vi "ANC300_Input.vi"(0 "ANC300 Communication Port In":refnum<visa-resource-name>, 1 "connection ID in":refnum<k5>, 2 "Axis":u8=1 min=1 max=7, 3 "ON / OFF":bool=TRUE, 4 "AC / DC":bool=TRUE, 5 "error in":T1, 7 "Time to wait [ms]":u32=200, 8 "set / get":bool=TRUE) -> (13 "command string":string, 14 "ANC300 Communication Port Out":refnum<visa-resource-name>, 15 "connection ID out":refnum<k5>, 16 "transfer ok":bool, 17 "ON / OFF":bool=TRUE, 18 "data out":string, 19 "error out":T1)   [LabVIEW 2022 SP3]
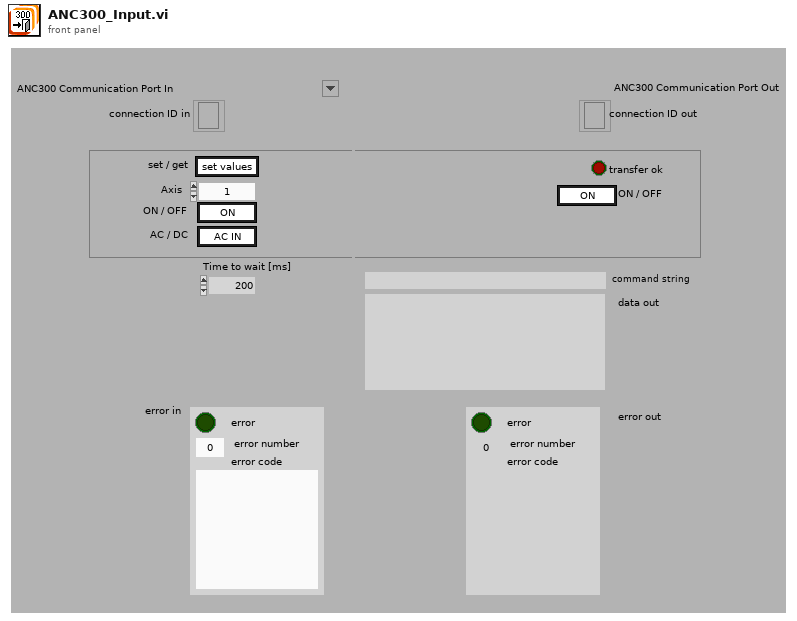
[diagram p1: front panel]
types:
  T1 = cluster{"error ":bool, "error number":i32, "error code":string}
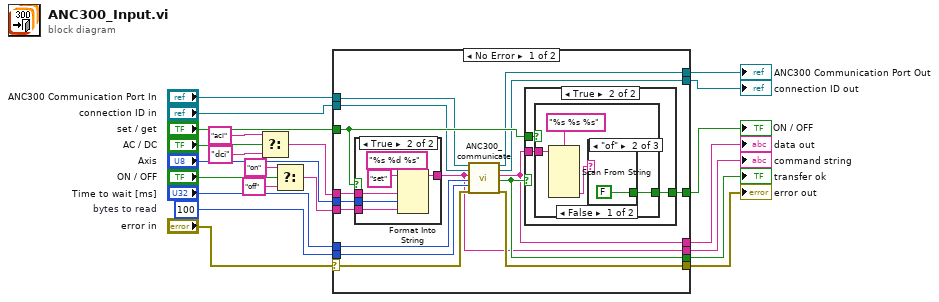
[diagram p0: block diagram]
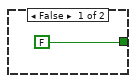
[diagram p2: hidden frame]
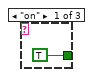
[diagram p3: hidden frame]
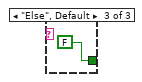
[diagram p4: hidden frame]
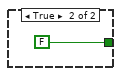
[diagram p5: hidden frame]
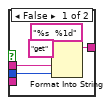
[diagram p6: hidden frame]
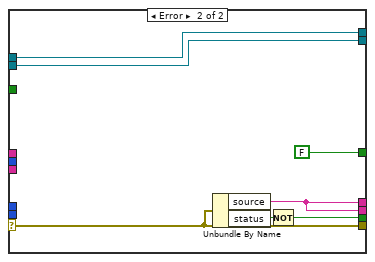
[diagram p7: hidden frame]
diagram:
  w17 = 100  # bytes to read
  n1 = Select(t="aci", s="AC / DC", f="dci") -> (s? t:f=w2:string)
  n2 = Select(t="on", s="ON / OFF", f="off") -> (s? t:f=w3:string)
  n3 = case shown="No Error" "error in" {
    selector: "error in" -> [w26 w66]
    tunnel: w2 -> [w38 _]
    tunnel: "Axis" -> [w37 _]
    tunnel: w3 -> [w36 _]
    tunnel: "set / get" -> [w35 _]
    tunnel: "ANC300 Communication Port In" -> [w34 w68]
    tunnel: "connection ID in" -> [w33 w67]
    tunnel: "Time to wait [ms]" -> [w32 _]
    tunnel: w17 -> [w31 _]
    tunnel: [w30 FALSE] -> w1
    tunnel: [w29 w66] -> w11
    tunnel: [w28 w68] -> w15
    tunnel: [w27 w67] -> w14
    tunnel: [w25 w64] -> w10
    tunnel: [w24 w63] -> w13
    tunnel: [w23 w63] -> w12
    frame No Error {
      n4 = case shown="True" w35 {
        tunnel: w37 -> [w51 w60]
        tunnel: w38 -> [w52 w59]
        tunnel: w36 -> [_ w58]
        tunnel: [w53 w57] -> w24
        frame False {
          n5 = Format Into String(format string="%s  %1d", initial string="get", w52, w51) -> (resulting string=w53:string)  [unwired: 1 in, 1 out]
        }
        frame True {
          n6 = Format Into String(format string="%s %d %s", initial string="set", w59, w60, w58) -> (resulting string=w57:string)  [unwired: 1 in, 1 out]
        }
      }
      n7 = call "ANC300_communicate.vi"("ANC300 Communication Port In"=w34, "connection ID in"=w33, "commando string"=w24, "Time to wait [ms]"=w32, "bytes to read"=w31, "error in"=w26) -> ("ANC300 Communication Port Out"=w28:refnum<visa-resource-name>, "connection ID out"=w27:refnum<k5>, "read data"=w23:string, "transfer ok"=w25:bool, "error out"=w29:T1)  [unwired: 9 in]
      n8 = case shown="True" w25 {
        tunnel: [FALSE w42] -> w30
        tunnel: w23 -> [_ w41]
        tunnel: w35 -> [_ w40]
        frame False {
        }
        frame True {
          n9 = case shown="False" w40 {
            tunnel: w41 -> [w45 _]
            tunnel: [w46 FALSE] -> w42
            frame False {
              n10 = Scan From String(format string="%s %s %s", input string=w45) -> (output 3=w43:string)  [unwired: 7 in, 3 out]
              n11 = case shown="\"of\"" w43 {
                tunnel: [TRUE FALSE FALSE] -> w46
                frame "on" {
                }
                frame "of" {
                }
                frame "Else", Default {
                }
              }
            }
            frame True {
            }
          }
        }
      }
    }
    frame Error {
      n12 = Unbundle By Name(w66) -> ("source"=w63:string, "status"=w65:bool)
      n13 = Not(x=w65) -> (.not. x?=w64:bool)
    }
  }
  "data out" <- w12
  "connection ID out" <- w14
  "error out" <- w11
  "command string" <- w13
  "transfer ok" <- w10
  "ANC300 Communication Port Out" <- w15
  "ON / OFF" <- w1
